vi "search data.vi"(9 "y":string, 11 "connection information":path) -> (3 "字符串":string)   [LabVIEW 2013]
uses:
  <vilib>/addons/database/Connection.llb/DB Tools Open Connec (Path).vi
  <vilib>/addons/database/NI_Database_API.lvlib
panel:
  out "子数组":string[](array[string])
  out "data":variant[][](array[variant])
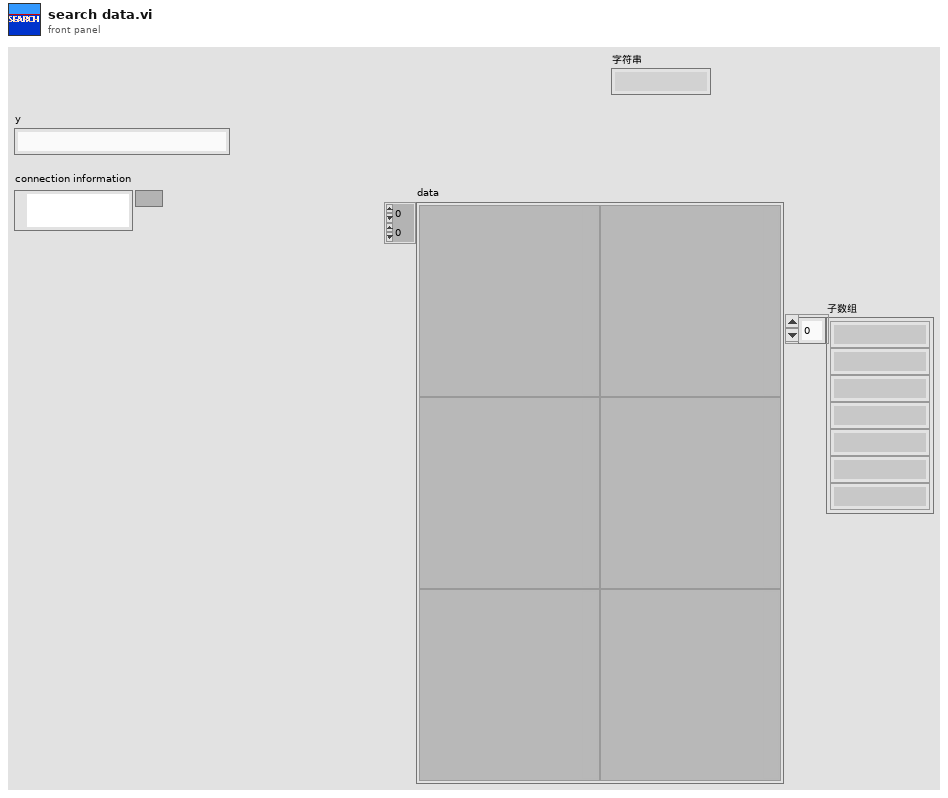
[diagram p1: front panel]
types:
  T1 = typedef "NI_Database_API.lvlib/Conn ObjectReference.ctl" = refnum<k1>
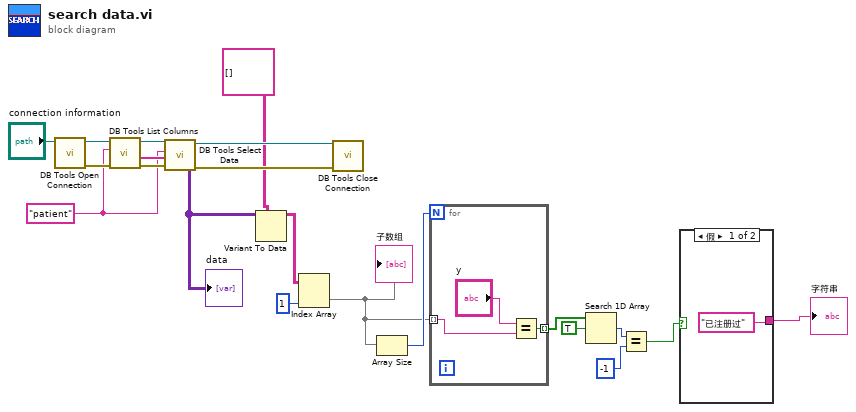
[diagram p0: block diagram]
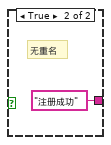
[diagram p2: hidden frame]
diagram:
  w15 = "patient"
  n1 = call-poly <vilib>:"DB Tools Open Connection.vi"("connection information"="connection information") -> ("error out"=w16:errorcluster, "connection reference"=w20:T1)  [unwired: 7 in]
  n2 = call <vilib>:"DB Tools List Columns.vi"("error in (no error)"=w16, "table"=w15, "connection reference"=w20) -> ("error out"=w17:errorcluster, "columns"=w18:string[], "connection reference out"=w19:T1)  [unwired: 1 in, 1 out]
  n3 = call <vilib>:"DB Tools Select Data.vi"("error in (no error)"=w17, "columns"=w18, "table"=w15, "connection reference"=w19) -> ("error out"=w13:errorcluster, "data"=w12:variant[][], "connection reference out"=w14:T1)  [unwired: 2 in]
  "data" <- w12
  n4 = Variant To Data(type=string[][] [], Variant=w12) -> (data=w10:string[][])  [unwired: 1 in, 1 out]
  n5 = Index Array(array=w10, index (col)=1 ("禁用的索引 (列)")) -> (element=w7:string[])  [unwired: 1 in]
  "子数组" <- w7
  n6 = call <vilib>:"DB Tools Close Connection.vi"("error in (no error)"=w13, "connection reference"=w14) -> ()  [unwired: 5 in, 1 out]
  n7 = Array Size(array=w7) -> (size(s)=w8:i32)
  n8 = for {
    N: w8 -> [_]
    tunnel: w7 -> [w24] mode=indexing
    tunnel: [w23] -> w6 mode=indexing
    n9 = Equal?(x="y", y=w24) -> (x = y?=w23:bool)
  }
  n10 = Search 1D Array(1D array=w6, element=TRUE ("元素")) -> (index of element=w3:i32)  [unwired: 1 in]
  n11 = Equal?(x=w3, y=-1) -> (x = y?=w2:bool)
  n12 = case shown="假" w2 {
    tunnel: ["已注册过" "注册成功"] -> w1
    frame False {
    }
    frame True {
      # "无重名"
    }
  }
  "字符串" <- w1
